vi "TestToJson.vi"(4 "erfolgreich":bool, 5 "Log":string, 6 "aktueller Test":string, 7 "reference":refnum<vi>, 8 "error in (no error)":errorcluster, 9 "Kommentar":string, 10 "Daten in":T1={"Report.lvclass"=refnum, "Norm"="", "last State"=enum."Initialize", "Norm ID"=0, "parameter"=[], "EMTestCWS500N.lvclass"=refnum, "CEG4500.lvclass"=refnum, "Tektronix RSA5106A.lvclass"=refnum, "erfolgreich"=FALSE, "log"="", "Kommentar"="", "Device Enum"=enum."emTestCWS500N", "Test Enum"=enum."HF-Felder", "debug"=FALSE, "tab"=enum."Hauptmenü", "ESD Pistol.lvclass"=refnum, "SubPnl Refnum"=refnum, "TabCtl Refnum"=refnum, "ButtonsEinblenden?"=FALSE, "VKey"=enum."ASCII"}, 11 "TestInterface in":refnum<class "TestInterface.lvclass">) -> (0 "error out":errorcluster, 3 "Daten out 2":T1={"Report.lvclass"=refnum, "Norm"="", "last State"=enum."Initialize", "Norm ID"=0, "parameter"=[], "EMTestCWS500N.lvclass"=refnum, "CEG4500.lvclass"=refnum, "Tektronix RSA5106A.lvclass"=refnum, "erfolgreich"=FALSE, "log"="", "Kommentar"="", "Device Enum"=enum."emTestCWS500N", "Test Enum"=enum."HF-Felder", "debug"=FALSE, "tab"=enum."Hauptmenü", "ESD Pistol.lvclass"=refnum, "SubPnl Refnum"=refnum, "TabCtl Refnum"=refnum, "ButtonsEinblenden?"=FALSE, "VKey"=enum."ASCII"})   [LabVIEW 2013, in "EMV-Test.lvlib"]
uses:
  EMV-Test.lvlib
  classes/Tests/TestInterface/TestInterface.lvclass
  classes/Devices/emTestCWS500N/EMTestCWS500N.lvclass
  classes/Devices/Tektronix RSA5106A/Tektronix RSA5106A.lvclass
  classes/Devices/CEG4500/CEG4500.lvclass
  classes/Datastructure/Report/Report.lvclass
  Main/controls/State.ctl
  classes/Devices/DeviceInterface/Devices.ctl
  classes/Tests/TestInterface/Tests.ctl
  Main/controls/Data.ctl
  vis/Tabs.ctl
  vis/ESD Pistol.lvclass
  <vilib>/event_ctls.llb/eventvkey.ctl
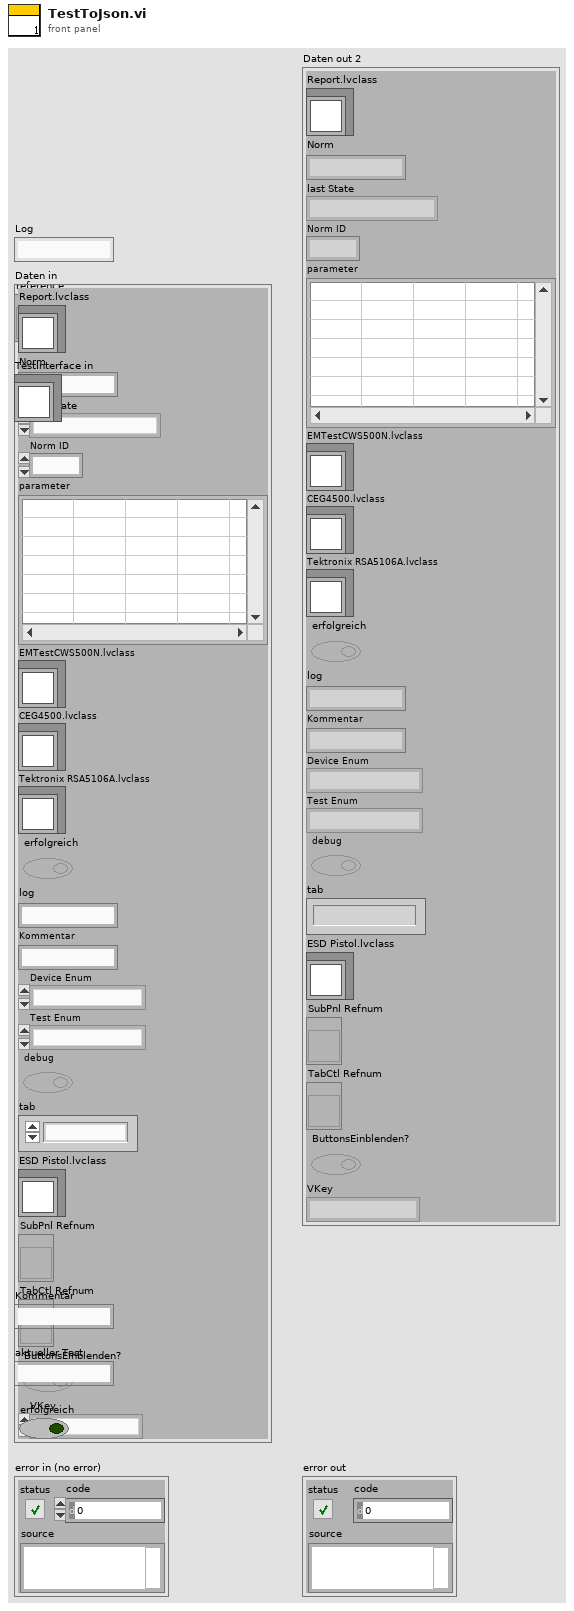
[diagram p1: front panel]
types:
  T1 = typedef "Data.ctl" = cluster{"Report.lvclass":refnum<class "Report.lvclass">, "Norm":string, "last State":T2, "Norm ID":i32, "parameter":string[][], "EMTestCWS500N.lvclass":refnum<class "EMTestCWS500N.lvclass">, "CEG4500.lvclass":refnum<class "CEG4500.lvclass">, "Tektronix RSA5106A.lvclass":refnum<class "Tektronix RSA5106A.lvclass">, "erfolgreich":bool, "log":string, "Kommentar":string, "Device Enum":T3, "Test Enum":T4, "debug":bool, "tab":T5, "ESD Pistol.lvclass":refnum<class "ESD Pistol.lvclass">, "SubPnl Refnum":refnum<vi>, "TabCtl Refnum":refnum<vi>, "ButtonsEinblenden?":bool, "VKey":T6}
  T2 = typedef "State.ctl" = enum16{"create Pdf", "edit Report", "load Report", "save Report", "do Test", "CDN Kalibrierung", "enter Report Parameters", "new Test", "Protokoll", "read Tree", "update Tree", "Fehler", "Initialize", "Wait for Event", "Exit"}
  T3 = typedef "Devices.ctl" = enum16{"unbekannt", "ESD Pistol", "Tektronix RSA5106A", "emTestCWS500N", "CEG-4500"}
  T4 = typedef "Tests.ctl" = enum16{"unbekannt", "Störaussendung", "Burst", "ESD", "Surge", "Spannungseinbruch", "HF-Felder"}
  T5 = typedef "Tabs.ctl" = enum32{"Hauptmenü", "Prüfbericht", "Einstellungen"}
  T6 = typedef "eventvkey.ctl" = enum16{"ASCII", "Enter", "Return", "Shift", "Ctrl", "Alt", "Cmd", "Opt", "Caps", "NumLock", "Clear", "Break", "Up", "Down", "Left", "Right", "Insert", "Delete", "Home", "End", "PageUp", "PageDown", "Escape", "Help", "Pause", "ScrollLock", "F1", "F2", "F3", "F4", "F5", "F6", "F7", "F8", "F9", "F10", "F11", "F12", "F13", "F14", "F15", "F16", "F17", "F18", "F19", "F20", "F21", "F22", "F23", "F24", "Play", "VolumeUp", "VolumeDown", "Mute", "Two Byte Char"}
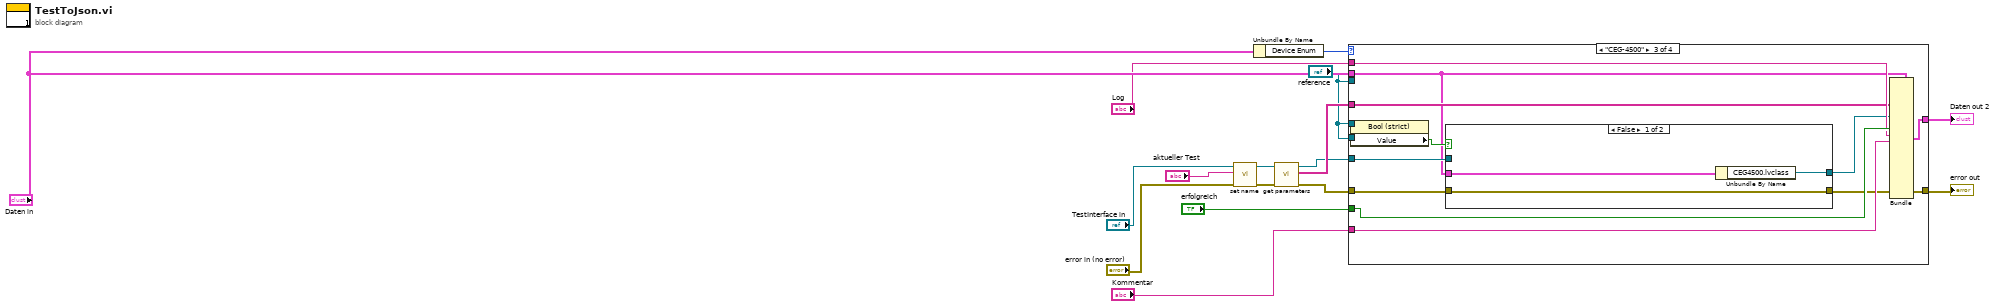
[diagram p0: block diagram]
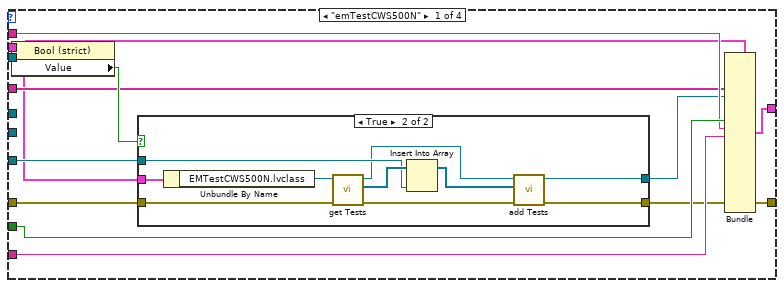
[diagram p2: hidden frame]
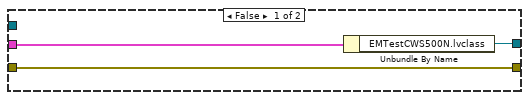
[diagram p3: hidden frame]
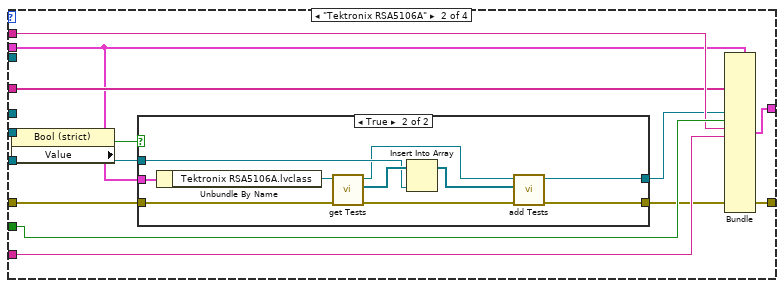
[diagram p4: hidden frame]
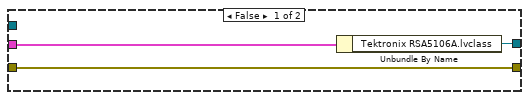
[diagram p5: hidden frame]
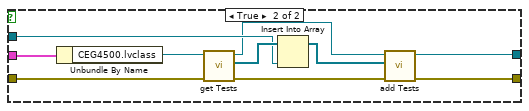
[diagram p6: hidden frame]
diagram:
  n1 = call-dynamic "set name.vi"("error in (no error)"="error in (no error)", "name"="aktueller Test", "TestInterface (Eingang)"="TestInterface in") -> ("error out"=w10:errorcluster, "TestInterface (Ausgang)"=w11:refnum<class "TestInterface.lvclass">)  [unwired: 7 in]
  n2 = Unbundle By Name("Daten in") -> ("Device Enum"=w14:T3)
  n3 = call-dynamic "get parameters.vi"("error in (no error)"=w10, "TestInterface (Eingang)"=w11) -> ("error out"=w4:errorcluster, "parameters"=w6:string[], "TestInterface (Ausgang)"=w3:refnum<class "TestInterface.lvclass">)  [unwired: 7 in]
  n4 = case shown="\"CEG-4500\"" w14 {
    tunnel: "erfolgreich" -> [w28 w53 w78 _]
    tunnel: "Log" -> [w27 w52 w77 _]
    tunnel: "Kommentar" -> [w26 w51 w76 _]
    tunnel: w3 -> [w24 w49 w74 _]
    tunnel: w4 -> [w23 w48 w73 w93]
    tunnel: [w22 w47 w72 w93] -> w5
    tunnel: [w19 w44 w71 w92] -> w15
    tunnel: w6 -> [w20 w46 w70 _]
    tunnel: "Daten in" -> [w18 w43 w68 w92]
    tunnel: "reference" -> [w17 _ _ _]
    tunnel: "reference" -> [_ w42 _ _]
    tunnel: "reference" -> [_ _ w67 _]
    frame "emTestCWS500N" {
      n5 = property class="Bool (strict)"(reference=w17) -> ("Value"=w25:bool)  [unwired: 1 in, 2 out]
      n6 = case shown="True" w25 {
        tunnel: w24 -> [_ w39]
        tunnel: w23 -> [w31 w35]
        tunnel: [w31 w34] -> w22
        tunnel: [w30 w33] -> w21
        tunnel: w18 -> [w29 w32]
        frame False {
          n7 = Unbundle By Name(w29) -> ("EMTestCWS500N.lvclass"=w30:refnum<class "EMTestCWS500N.lvclass">)
        }
        frame True {
          n8 = Unbundle By Name(w32) -> ("EMTestCWS500N.lvclass"=w41:refnum<class "EMTestCWS500N.lvclass">)
          n9 = call-dynamic "get Tests.vi"("error in (no error)"=w35, "DeviceInterface (Eingang)"=w41) -> ("error out"=w36:errorcluster, "Tests"=w40:refnum<class "TestInterface.lvclass">[], "DeviceInterface (Ausgang)"=w37:refnum<class "EMTestCWS500N.lvclass">)  [unwired: 7 in]
          n10 = Insert Into Array(array=w40, new element=w39) -> (w38:refnum<class "TestInterface.lvclass">[])  [unwired: 1 in]
          n11 = call-dynamic "add Tests.vi"("error in (no error)"=w36, "Tests"=w38, "DeviceInterface (Eingang)"=w37) -> ("error out"=w34:errorcluster, "DeviceInterface (Ausgang)"=w33:refnum<class "EMTestCWS500N.lvclass">)  [unwired: 7 in]
        }
      }
      n12 = Bundle(cluster=w18, "parameter"=w20, "EMTestCWS500N.lvclass"=w21, "erfolgreich"=w28, "log"=w27, "Kommentar"=w26) -> (w19:T1)  [unwired: 15 in]
    }
    frame "Tektronix RSA5106A" {
      n13 = property class="Bool (strict)"(reference=w42) -> ("Value"=w50:bool)  [unwired: 1 in, 2 out]
      n14 = case shown="True" w50 {
        tunnel: w49 -> [_ w64]
        tunnel: w48 -> [w56 w60]
        tunnel: [w56 w59] -> w47
        tunnel: [w55 w58] -> w45
        tunnel: w43 -> [w54 w57]
        frame False {
          n15 = Unbundle By Name(w54) -> ("Tektronix RSA5106A.lvclass"=w55:refnum<class "Tektronix RSA5106A.lvclass">)
        }
        frame True {
          n16 = Unbundle By Name(w57) -> ("Tektronix RSA5106A.lvclass"=w66:refnum<class "Tektronix RSA5106A.lvclass">)
          n17 = call-dynamic "get Tests.vi"("error in (no error)"=w60, "DeviceInterface (Eingang)"=w66) -> ("error out"=w61:errorcluster, "Tests"=w65:refnum<class "TestInterface.lvclass">[], "DeviceInterface (Ausgang)"=w62:refnum<class "Tektronix RSA5106A.lvclass">)  [unwired: 7 in]
          n18 = Insert Into Array(array=w65, new element=w64) -> (w63:refnum<class "TestInterface.lvclass">[])  [unwired: 1 in]
          n19 = call-dynamic "add Tests.vi"("error in (no error)"=w61, "Tests"=w63, "DeviceInterface (Eingang)"=w62) -> ("error out"=w59:errorcluster, "DeviceInterface (Ausgang)"=w58:refnum<class "Tektronix RSA5106A.lvclass">)  [unwired: 7 in]
        }
      }
      n20 = Bundle(cluster=w43, "parameter"=w46, "Tektronix RSA5106A.lvclass"=w45, "erfolgreich"=w53, "log"=w52, "Kommentar"=w51) -> (w44:T1)  [unwired: 15 in]
    }
    frame "CEG-4500" {
      n21 = property class="Bool (strict)"(reference=w67) -> ("Value"=w75:bool)  [unwired: 1 in, 2 out]
      n22 = case shown="False" w75 {
        tunnel: w74 -> [_ w89]
        tunnel: w73 -> [w80 w85]
        tunnel: [w80 w84] -> w72
        tunnel: [w81 w83] -> w69
        tunnel: w68 -> [w79 w82]
        frame False {
          n23 = Unbundle By Name(w79) -> ("CEG4500.lvclass"=w81:refnum<class "CEG4500.lvclass">)
        }
        frame True {
          n24 = Unbundle By Name(w82) -> ("CEG4500.lvclass"=w91:refnum<class "CEG4500.lvclass">)
          n25 = call-dynamic "get Tests.vi"("error in (no error)"=w85, "DeviceInterface (Eingang)"=w91) -> ("error out"=w86:errorcluster, "Tests"=w90:refnum<class "TestInterface.lvclass">[], "DeviceInterface (Ausgang)"=w87:refnum<class "CEG4500.lvclass">)  [unwired: 7 in]
          n26 = Insert Into Array(array=w90, new element=w89) -> (w88:refnum<class "TestInterface.lvclass">[])  [unwired: 1 in]
          n27 = call-dynamic "add Tests.vi"("error in (no error)"=w86, "Tests"=w88, "DeviceInterface (Eingang)"=w87) -> ("error out"=w84:errorcluster, "DeviceInterface (Ausgang)"=w83:refnum<class "CEG4500.lvclass">)  [unwired: 7 in]
        }
      }
      n28 = Bundle(cluster=w68, "parameter"=w70, "CEG4500.lvclass"=w69, "erfolgreich"=w78, "log"=w77, "Kommentar"=w76) -> (w71:T1)  [unwired: 15 in]
    }
    frame "unbekannt" {
    }
  }
  "Daten out 2" <- w15
  "error out" <- w5
